vi "PAQ_BIN_Read_Index.vi"(8 "error in (no error)":errorcluster, 10 "TableName":string, 11 "Path":path) -> (0 "error out":errorcluster, 3 "TimeStamps":T1(array[cluster]))   [LabVIEW 2020, in "Sgraph_lib_V1.lvlib" / "DBAL-BIN.lvclass"]
doc: "Read the index file of a specific layer on disk"
uses:
  DBAL-BIN.lvclass
panel:
  out "Cluster":T2
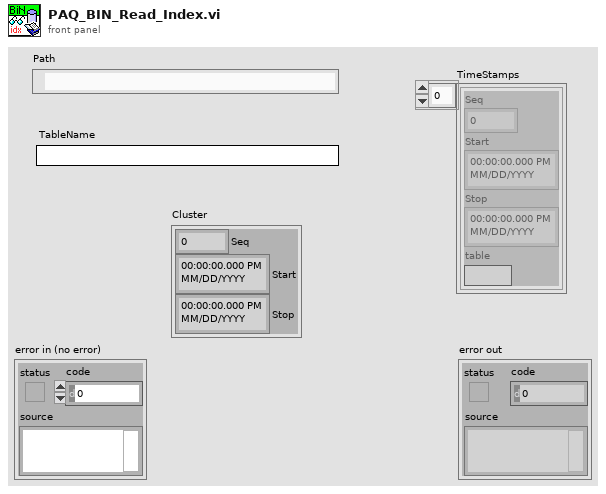
[diagram p1: front panel]
types:
  T1 = cluster{"Seq":i32, "Start":timestamp, "Stop":timestamp, "table":string}[]
  T2 = cluster{"Seq":dbl, "Start":timestamp, "Stop":timestamp}
  T3 = cluster{"Seq":i32, "Start":timestamp, "Stop":timestamp, "Table":string}
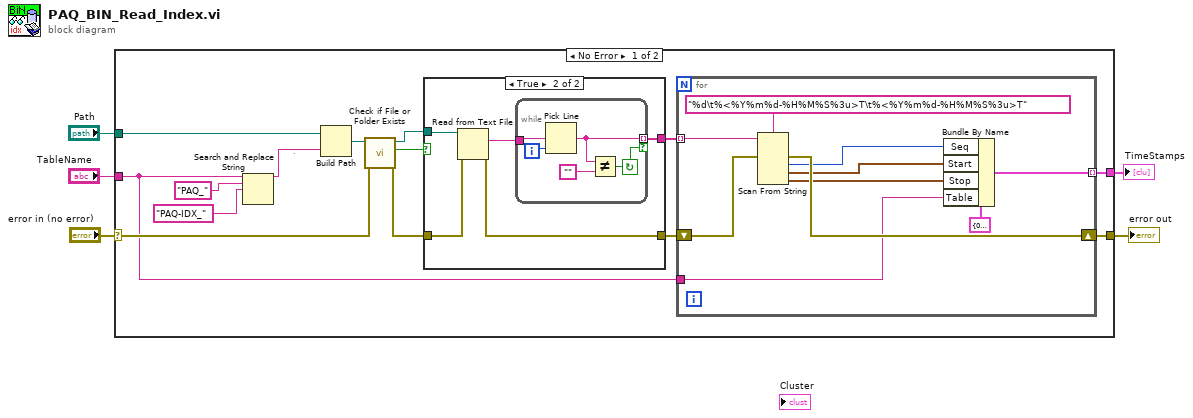
[diagram p0: block diagram]
diagram:
  n1 = case shown="No Error" "error in (no error)" {
    selector: "error in (no error)" -> [w15 w41]
    tunnel: [w7 w41] -> w4
    tunnel: "TableName" -> [w6 _]
    tunnel: "Path" -> [w17 _]
    tunnel: [w10 _] -> w1
    frame No Error {
      # "`"
      n2 = Search and Replace String(input string=w6, search string="PAQ_", replace string="PAQ-IDX_" ("search string")) -> (result string=w9:string)  [unwired: 5 in, 3 out]
      n3 = Build Path(base path=w17, name or relative path=w9) -> (appended path=w16:path)
      n4 = call <vilib>:"Check if File or Folder Exists.vi"("error in (no error)"=w15, "path"=w16) -> ("error out"=w12:errorcluster, "file or folder exists?"=w14:bool, "dup path"=w13:path)  [unwired: 7 in]
      n5 = case shown="True" w14 {
        tunnel: w13 -> [_ w35]
        tunnel: w12 -> [w30 w34]
        tunnel: [w30 w33] -> w8
        tunnel: [_ w31] -> w11
        frame False {
        }
        frame True {
          n6 = Read from Text File(file (use dialog)=w35, error in=w34) -> (text=w32:string, error out=w33:errorcluster)  [unwired: 2 in, 2 out]
          n7 = while {
            tunnel: w32 -> [w40]
            tunnel: [w38] -> w31 mode=indexing if=w36
            i -> [w39]
            stop <- w36 continue-if-true
            n8 = Pick Line(multi-line string=w40, line index=w39) -> (output string=w38:string)  [unwired: 1 in]
            n9 = Not Equal?(x=w38, y="") -> (x != y?=w36:bool)
          }
        }
      }
      n10 = for {
        tunnel: w11 -> [w29] mode=indexing
        tunnel: [w25] -> w10 mode=indexing
        shift-right: [w26] -> w7
        shift-left: w8 -> [w27]
        tunnel: w6 -> [w20]
        n11 = Scan From String(format string="%d\t%<%Y%m%d-%H%M%S%3u>T\t%<%Y%m%d-%H%M%S%3u>T", input string=w29, error in=w27) -> (error out=w26:errorcluster, output 1=w21:i32, output 2=w22:timestamp, output 3=w23:timestamp)  [unwired: 4 in, 2 out]
        n12 = Bundle By Name(cluster=T3 {"Seq"=0, "Start"=timestamp(0 s since 1904-01-01), "Stop"=timestamp(0 s since 1904-01-01), "Table"=""} ("Cluster"), "Seq"=w21, "Start"=w22, "Stop"=w23, "Table"=w20) -> (w25:T3)
      }
    }
    frame Error {
    }
  }
  "error out" <- w4
  "TimeStamps" <- w1
